vi "setFPGAReference.vi"(10 "FPGAReference":refnum<k20>, 11 "FPGATelemetry in":refnum<class "FPGATelemetry.lvclass">) -> (3 "FPGATelemetry out":refnum<class "FPGATelemetry.lvclass">)   [LabVIEW 2015, in "FPGATelemetry.lvclass"]
uses:
  FPGATelemetry.lvclass
  FPGATelemetry.lvclass/FPGATelemetry.ctl
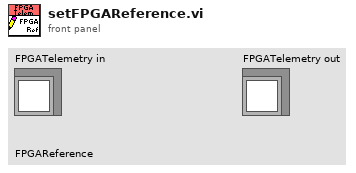
[diagram p1: front panel]
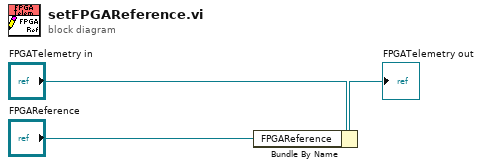
[diagram p0: block diagram]
diagram:
  n1 = Bundle By Name(cluster="FPGATelemetry in", "FPGAReference"="FPGAReference") -> (→"FPGATelemetry out":refnum<class "FPGATelemetry.lvclass">)
